vi "Check R Create Dir.vi"(11 "File Path":path=path "C:/Documents and Settings/muddaspr/My Documents") -> (3 "Dir Path":path)   [LabVIEW 2018]
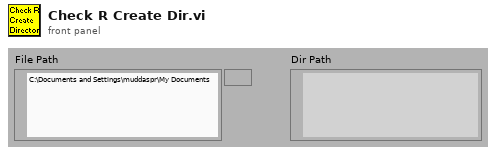
[diagram p1: front panel]
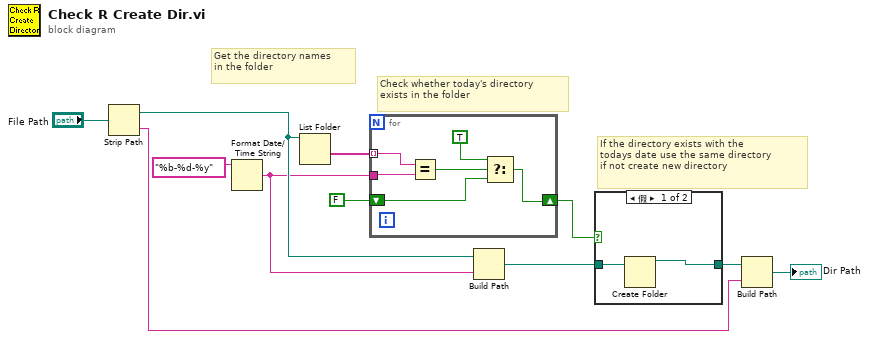
[diagram p0: block diagram]
diagram:
  # "If the directory exists with the\ntodays date use the same directory\nif not create new directory"
  # "Check whether today's directory\nexists in the folder"
  # "Get the directory names\nin the folder"
  n1 = Strip Path(path="File Path") -> (stripped path=w4:path, name=w1:string)
  n2 = Format Date/Time String(time format string (%c)="%b-%d-%y") -> (date/time string=w3:string)  [unwired: 2 in]
  n3 = List Folder(path=w4) -> (folder names=w8:string[])  [unwired: 3 in, 3 out]
  n4 = for {
    tunnel: w8 -> [w17] mode=indexing
    tunnel: w3 -> [w16]
    shift-right: [w14] -> w6
    shift-left: FALSE -> [w13]
    n5 = Equal?(x=w17, y=w16) -> (x = y?=w15:bool)
    n6 = Select(t=TRUE, s=w15, f=w13) -> (s? t:f=w14:bool)
  }
  n7 = Build Path(base path=w4, name or relative path=w3) -> (appended path=w9:path)
  n8 = case shown="假" w6 {
    tunnel: w9 -> [w19 w20]
    tunnel: [w18 w20] -> w5
    frame False {
      n9 = Create Folder(path (use dialog)=w19) -> (created path=w18:path)  [unwired: 2 in, 2 out]
    }
    frame True {
    }
  }
  n10 = Build Path(base path=w5, name or relative path=w1) -> (appended path=→"Dir Path":path)
